vi "PCC_2act_acq.vi"() -> ()   [LabVIEW 2020]
uses:
  C:/Users/quic2/Desktop/DirectUQDLabviewCode/Kinesis/Thorlabs.MotionControl.Controls.dll
  Kinesis/Thorlabs.MotionControl.Controls.dll
  C:/Program Files/Dotfast Consulting/Timetag Explorer 2.26/ttInterface.dll
  Program Files/Dotfast Consulting/Timetag Explorer 2.26/ttInterface.dll
  C:/Users/quic2/Desktop/DirectUQDLabviewCode/Kinesis/ThorLabs.MotionControl.KCube.DCServoCLI.dll
  Kinesis/ThorLabs.MotionControl.KCube.DCServoCLI.dll
  C:/Users/quic2/Desktop/DirectUQDLabviewCode/Kinesis/Thorlabs.MotionControl.KCube.StepperMotorCLI.dll
  Kinesis/Thorlabs.MotionControl.KCube.StepperMotorCLI.dll
  <vilib>/Utility/file.llb/Write Delimited Spreadsheet (string).vi
panel:
  out "x*y":i32=524580565 format="%.3p"
  out "Header":string[](array[string])=["Time Counter (5ns)", "R", "S1", "S2", "RvS1b", "RvS1p", "RvS2b", "RvS2p", "S1pvS2p", "S1bvS2b", "S1bvS2p", "S1pvS2b", "RvS1pvS2p", "RvS1bvS2b"]
  out "R Singles\n Rate (Hz)":u32=294126 format="%.2p"
  out "Horizontal S1\n singles Rate (Hz)":u32=5 format="%.2p"
  out "Vertical S2 \nSingles Rate (Hz)":u32=5 format="%.2p"
  in  "Repetitions":i32=5
  in  "Acquisition \nTime (s)":dbl=0.5
  in  "V  Zero Error":dbl=7.0 format="%#_13g"
  in  "H Zero Error":dbl=7.5 format="%#_13g"
  in  "HWP_ZeroError":dbl=15.0 format="%#_13g"
  out "Current HWP Angle":dbl=15.0
  out "V centroid Singles":dbl=6.986141506451791
  out "H centroid Singles":dbl=7.447438431946241
  out "V Singles":dbl=6.950874322723666 format="%.4e"
  out "H Singles":dbl=7.7419281256167665 format="%.4e"
  in  "Folder":path=path "D:/PCC/2021/3_March/directUQD/6thMarch/RawFileTest/Test5"
  in  "# of Beam Scan":i32=1
  out "V Position":dbl=7.25
  out "H Position":dbl=9.0
  in  "stop":bool
  out "HWP #Iterations":dbl
  out "V # Iterations":dbl=60.0
  out "H #Iterations":dbl=60.0
  in  "HWP_ Stop":dbl=20.0 min=0.0 max=359.0
  in  "HWP_Step":dbl=10.0 min=1e-05 max=359.0
  in  "V Final Position":dbl=7.25 min=0.0 max=25.0
  in  "V Step":dbl=0.05 min=1e-10 max=15.0
  in  "H Final Position":dbl=9.0 min=0.0 max=25.0
  in  "H Step":dbl=0.05 min=1e-10 max=15.0
  in  "V Initial Position":dbl=4.0 min=0.0 max=25.0
  in  "HWP_Start":dbl=15.0 min=0.0 max=359.0
  in  "HWP_post":refnum<k24>(container)
  in  "H Initial Position":dbl=5.75 min=0.0 max=25.0
  in  "Actuator Vertical":refnum<k24>(container)
  in  "Actuator Horizontal":refnum<k24>(container)
  out "Waveform Chart":T1(graph)
  out "Time per Pos":dbl=2.5
  out "Array":i32[](array[numeric])=[844176, 4, 12, 0, 0, 0, 0, 0, 0, 0, 0, 0, 0]
  in  "Ctw(ns)":dbl=2.0
  in  "S2b":u8=10
  in  "S2p":u8=9
  in  "S1b":u8=8
  in  "S1p":u8=7
  in  "R":u8=5
  in  "Ch Array":u8[](array[numeric])=[5, 7, 8, 9, 10] caption="Ch"
  in  "Ch Delay (ns)":dbl[](array[numeric])=[120.0, 11.0, 86.0, 7.5, 82.5]
  # "FOLDER PATH"
  # "HORIZONTAL ACTUATOR"
  # "VERTICAL ACTUATOR"
  # "POST-SELECTION HWP"
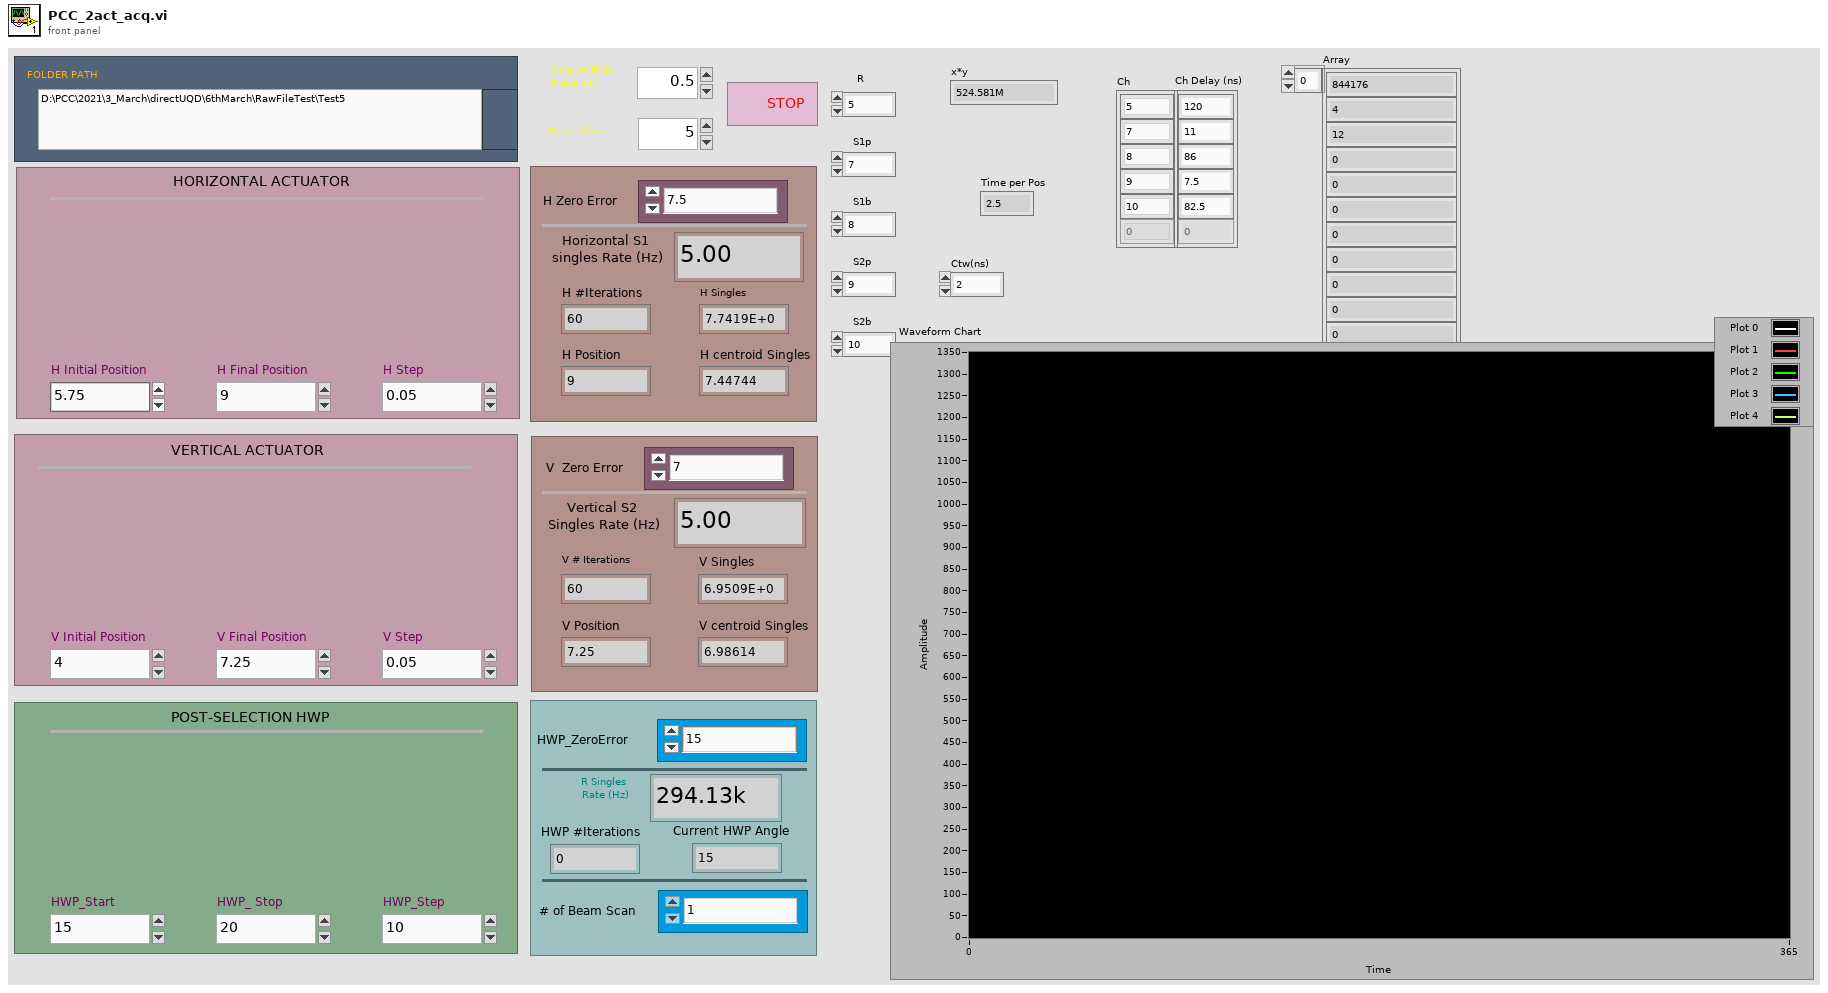
[diagram p1: front panel]
types:
  T1 = cluster{"[0]":dbl, "[1]":dbl, "[2]":dbl, "[3]":dbl, "[4]":dbl, "[5]":dbl, "[6]":dbl, "[7]":dbl, "[8]":dbl}
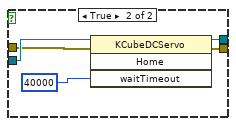
[diagram p3: hidden frame]
diagram:
  # "We want 3 singles\n4 coincidences(peak)\n4 coincidences(BG)\n\nLogic 16 channels\nWe neeed 4+4+3 =11\n\n\nLogic has no per ch delay\nThey must be added in physical channel\n\nSo we need at least 5 physical Chanel\n1 for ref (100)\n1 for H S (delay for peak, 5 )\n1 for HS (delay BG, 75)\n(split the sma into 2 anc connect\nSame signal in both channels)"
  n1 = flat-sequence {
    tunnel: [w110] -> w30
    tunnel: [w109] -> w29
    tunnel: w30 -> [w125]
    tunnel: w29 -> [w124]
    tunnel: [w132] -> w86
    tunnel: [w131] -> w85
    tunnel: [w130] -> w78
    tunnel: [w129] -> w77
    tunnel: w86 -> [w154]
    tunnel: w85 -> [w153]
    tunnel: [w154] -> w83
    tunnel: [w153] -> w81
    tunnel: [w152] -> w79
    tunnel: w78 -> [w151]
    tunnel: w77 -> [w150]
    tunnel: [w151] -> w70
    tunnel: [w150] -> w63
    tunnel: [w149] -> w60
    tunnel: [w148] -> w59
    tunnel: [w147] -> w19
    tunnel: [w181] -> w84
    tunnel: w83 -> [w181]
    tunnel: [w180] -> w82
    tunnel: w81 -> [w180]
    tunnel: [w179] -> w80
    tunnel: w79 -> [w179]
    tunnel: [w178] -> w71
    tunnel: w70 -> [w178]
    tunnel: [w177] -> w64
    tunnel: w63 -> [w177]
    tunnel: w60 -> [w176]
    tunnel: w59 -> [w175]
    tunnel: [w176] -> w53
    tunnel: [w175] -> w45
    tunnel: [w174] -> w38
    tunnel: [w173] -> w31
    tunnel: [w172] -> w20
    tunnel: w19 -> [w172]
    tunnel: [w171] -> w18
    tunnel: [w170] -> w17
    tunnel: [w209] -> w108
    tunnel: [w211] -> w107
    tunnel: [w210] -> w106
    tunnel: [w209] -> w92
    tunnel: w84 -> [w202]
    tunnel: w82 -> [w201]
    tunnel: w80 -> [w200]
    tunnel: [w208] -> w72
    tunnel: w71 -> [w208]
    tunnel: [w207] -> w65
    tunnel: w64 -> [w207]
    tunnel: [w206] -> w54
    tunnel: w53 -> [w206]
    tunnel: [w205] -> w46
    tunnel: w45 -> [w205]
    tunnel: [w204] -> w39
    tunnel: w38 -> [w204]
    tunnel: [w203] -> w32
    tunnel: w31 -> [w203]
    tunnel: [w202] -> w27
    tunnel: [w201] -> w25
    tunnel: w20 -> [w199]
    tunnel: w18 -> [w198]
    tunnel: w17 -> [w197]
    tunnel: [w200] -> w15
    tunnel: [w199] -> w13
    tunnel: [w198] -> w11
    tunnel: [w197] -> w9
    tunnel: w108 -> [w247]
    tunnel: w107 -> [w246]
    tunnel: w106 -> [w231]
    tunnel: [w236] -> w105
    tunnel: [w235] -> w104
    tunnel: [w230] -> w99
    tunnel: w92 -> [w229]
    tunnel: [w229] -> w91
    tunnel: [w228] -> w73
    tunnel: w72 -> [w228]
    tunnel: [w227] -> w66
    tunnel: w65 -> [w227]
    tunnel: [w226] -> w55
    tunnel: w54 -> [w226]
    tunnel: [w225] -> w47
    tunnel: w46 -> [w225]
    tunnel: [w224] -> w40
    tunnel: w39 -> [w224]
    tunnel: [w223] -> w33
    tunnel: w32 -> [w223]
    tunnel: [w222] -> w28
    tunnel: w27 -> [w222]
    tunnel: [w221] -> w26
    tunnel: w25 -> [w221]
    tunnel: [w220] -> w16
    tunnel: w15 -> [w220]
    tunnel: [w219] -> w14
    tunnel: w13 -> [w219]
    tunnel: [w218] -> w12
    tunnel: w11 -> [w218]
    tunnel: [w217] -> w10
    tunnel: w9 -> [w217]
    tunnel: w105 -> [w272]
    tunnel: w104 -> [w271]
    tunnel: [w272] -> w103
    tunnel: [w271] -> w102
    tunnel: [w270] -> w101
    tunnel: [w269] -> w100
    tunnel: w99 -> [w269]
    tunnel: w91 -> [w268]
    tunnel: [w268] -> w90
    tunnel: [w267] -> w74
    tunnel: w73 -> [w267]
    tunnel: [w266] -> w67
    tunnel: w66 -> [w266]
    tunnel: [w265] -> w56
    tunnel: w55 -> [w265]
    tunnel: [w264] -> w48
    tunnel: w47 -> [w264]
    tunnel: [w263] -> w41
    tunnel: w40 -> [w263]
    tunnel: [w262] -> w34
    tunnel: w33 -> [w262]
    tunnel: w28 -> [w261]
    tunnel: w26 -> [w260]
    tunnel: [w261] -> w23
    tunnel: [w260] -> w21
    tunnel: w16 -> [w257]
    tunnel: w14 -> [w256]
    tunnel: w12 -> [w259]
    tunnel: w10 -> [w258]
    tunnel: [w259] -> w7
    tunnel: [w258] -> w5
    tunnel: [w257] -> w3
    tunnel: [w256] -> w1
    tunnel: w103 -> [w328]
    tunnel: w102 -> [w327]
    tunnel: w101 -> [w329]
    tunnel: w100 -> [w326]
    tunnel: [w329] -> w98
    tunnel: [w321] -> w97
    tunnel: [w320] -> w96
    tunnel: [w305] -> w95
    tunnel: w90 -> [w319]
    tunnel: [w319] -> w89
    tunnel: [w304] -> w87
    tunnel: [w317] -> w75
    tunnel: w74 -> [w317]
    tunnel: [w316] -> w68
    tunnel: w67 -> [w316]
    tunnel: [w315] -> w57
    tunnel: w56 -> [w315]
    tunnel: [w314] -> w49
    tunnel: w48 -> [w314]
    tunnel: [w313] -> w42
    tunnel: w41 -> [w313]
    tunnel: [w312] -> w35
    tunnel: w34 -> [w312]
    tunnel: [w311] -> w24
    tunnel: w23 -> [w311]
    tunnel: [w310] -> w22
    tunnel: w21 -> [w310]
    tunnel: [w309] -> w8
    tunnel: w7 -> [w309]
    tunnel: [w308] -> w6
    tunnel: w5 -> [w308]
    tunnel: [w307] -> w4
    tunnel: w3 -> [w307]
    tunnel: [w306] -> w2
    tunnel: w1 -> [w306]
    tunnel: w98 -> [w347]
    tunnel: w97 -> [w349]
    tunnel: w96 -> [w348]
    tunnel: w95 -> [w346]
    tunnel: [w345] -> w94
    tunnel: [w344] -> w93
    tunnel: w89 -> [w343]
    tunnel: [w343] -> w88
    tunnel: w87 -> [w342]
    tunnel: [w341] -> w76
    tunnel: w75 -> [w341]
    tunnel: [w340] -> w69
    tunnel: w68 -> [w340]
    tunnel: [w339] -> w58
    tunnel: w57 -> [w339]
    tunnel: [w338] -> w50
    tunnel: w49 -> [w338]
    tunnel: [w337] -> w43
    tunnel: w42 -> [w337]
    tunnel: [w336] -> w36
    tunnel: w35 -> [w336]
    tunnel: w24 -> [w335]
    tunnel: w22 -> [w334]
    tunnel: w8 -> [w333]
    tunnel: w6 -> [w332]
    tunnel: w4 -> [w331]
    tunnel: w2 -> [w330]
    tunnel: w94 -> [w608]
    tunnel: w93 -> [w607]
    tunnel: w88 -> [w606]
    tunnel: w76 -> [w604]
    tunnel: w69 -> [w603]
    tunnel: [w604] -> w62
    tunnel: [w603] -> w61
    tunnel: w58 -> [w602]
    tunnel: [w602] -> w52
    tunnel: [w601] -> w51
    tunnel: w50 -> [w601]
    tunnel: [w600] -> w44
    tunnel: w43 -> [w600]
    tunnel: [w599] -> w37
    tunnel: w36 -> [w599]
    tunnel: w62 -> [w612]
    tunnel: w61 -> [w609]
    tunnel: w52 -> [w616]
    tunnel: w51 -> [w613]
    tunnel: w44 -> [w618]
    tunnel: w37 -> [w617]
    frame #0 {
    }
    frame #1 {
      # "Calculate Iterations"
      n2 = local read "V Initial Position"() -> (w113:dbl)
      n3 = local read "V Final Position"() -> (w114:dbl)
      n4 = local read "H Initial Position"() -> (w117:dbl)
      n5 = local read "H Final Position"() -> (w118:dbl)
      n6 = local read "V Step"() -> (w111:dbl)
      n7 = local read "HWP_ Stop"() -> (w123:dbl)
      n8 = local read "HWP_Step"() -> (w120:dbl)
      n9 = local read "H Step"() -> (w116:dbl)
      n10 = local read "HWP_Start"() -> (w122:dbl)
      n11 = Subtract(x=w123, y=w122) -> (x-y=w121:dbl)
      n12 = Subtract(x=w114, y=w113) -> (x-y=w112:dbl)
      n13 = Subtract(x=w118, y=w117) -> (x-y=w115:dbl)
      n14 = Quotient & Remainder(x=w121, y=w120) -> (floor(x/y)=w119:dbl)  [unwired: 1 out]
      n15 = Quotient & Remainder(x=w112, y=w111) -> (floor(x/y)=w109:dbl)  [unwired: 1 out]
      n16 = Quotient & Remainder(x=w115, y=w116) -> (floor(x/y)=w110:dbl)  [unwired: 1 out]
      n17 = local write "HWP #Iterations"(w119) -> ()
      n18 = local write "V # Iterations"(w109) -> ()
      n19 = local write "H #Iterations"(w110) -> ()
    }
    frame #2 {
      # "Check if # iterations are same for H and V actuators"
      n20 = Not Equal?(x=w125, y=w124) -> (x != y?=w126:bool)
      n21 = case shown="True" w126 {
        frame False {
        }
        frame True {
          n22 = call "Display Message to User"() -> ("OK"=w127:bool)  [unwired: 10 in, 1 out]
          n23 = Stop(stop? (T)=w127) -> ()
        }
      }
    }
    frame #3 {
      # "Create HWP_post"
      n24 = property class="KCubeDCServoControl"(reference="HWP_post", "SerialNumber"="27503775") -> (reference out=w138:refnum<k24>, error out=w137:errorcluster)  [unwired: 1 in]
      n25 = invoke class="KCubeDCServoControl" method="CreateDevice"(reference=w138, error in=w137) -> (reference out=w135:refnum<k24>, error out=w136:errorcluster)  [unwired: 1 in, 1 out]
      n26 = property class="KCubeDCServoControl"(reference=w135, error in=w136) -> (reference out=w130:refnum<k24>, error out=w129:errorcluster, "Device"=w134:refnum<k24>)
      n27 = case shown="False" FALSE {
        tunnel: w134 -> [w141 w146]
        tunnel: [w141 w144] -> w132
        tunnel: [w140 w143] -> w131
        tunnel: w129 -> [w140 w142]
        frame False {
        }
        frame True {
          n28 = invoke class="KCubeDCServo" method="Home"(reference=w146, error in=w142, "waitTimeout"=40000) -> (reference out=w144:refnum<k24>, error out=w143:errorcluster)  [unwired: 1 in, 2 out]
        }
      }
    }
    frame #4 {
      # "Create H-Actuator"
      n29 = property class="KCubeStepperControl"(reference="Actuator Horizontal", "SerialNumber"="26002814") -> (reference out=w158:refnum<k24>, error out=w159:errorcluster)  [unwired: 1 in]
      n30 = invoke class="KCubeStepperControl" method="CreateDevice"(reference=w158, error in=w159) -> (reference out=w161:refnum<k24>, error out=w160:errorcluster)  [unwired: 1 in, 1 out]
      n31 = property class="KCubeStepperControl"(reference=w161, error in=w160) -> (reference out=w149:refnum<k24>, error out=w148:errorcluster, "Device"=w162:refnum<k24>)
      n32 = case shown="True" FALSE {
        tunnel: w162 -> [w164 w169]
        tunnel: w148 -> [w163 w167]
        tunnel: [w163 w166] -> w147
        tunnel: [w164 w165] -> w152
        frame False {
        }
        frame True {
          n33 = invoke class="KCubeStepper" method="Home"(reference=w169, error in=w167, "waitTimeout"=36000) -> (reference out=w165:refnum<k24>, error out=w166:errorcluster)  [unwired: 1 in, 2 out]
        }
      }
    }
    frame #5 {
      # "Create V-Actuator"
      n34 = property class="KCubeStepperControl"(reference="Actuator Vertical", "SerialNumber"="26001200") -> (reference out=w189:refnum<k24>, error out=w188:errorcluster)  [unwired: 1 in]
      n35 = invoke class="KCubeStepperControl" method="CreateDevice"(reference=w189, error in=w188) -> (reference out=w186:refnum<k24>, error out=w187:errorcluster)  [unwired: 1 in, 1 out]
      n36 = property class="KCubeStepperControl"(reference=w186, error in=w187) -> (reference out=w174:refnum<k24>, error out=w173:errorcluster, "Device"=w185:refnum<k24>)
      n37 = case shown="True" FALSE {
        tunnel: w185 -> [w191 w196]
        tunnel: w173 -> [w190 w194]
        tunnel: [w190 w193] -> w170
        tunnel: [w191 w192] -> w171
        frame False {
        }
        frame True {
          n38 = invoke class="KCubeStepper" method="Home"(reference=w196, error in=w194, "waitTimeout"=36000) -> (reference out=w192:refnum<k24>, error out=w193:errorcluster)  [unwired: 1 in, 2 out]
        }
      }
    }
    frame #6 {
      # "Create UQD TimeTag Interface"
      n39 = constructor class="TTInterface"() -> (reference out=w216:refnum<k24>, error out=w215:errorcluster)  [unwired: 3 in, 1 out]
      n40 = invoke class="TTInterface" method="Open"(reference=w216, error in=w215, "nr"=1) -> (reference out=w212:refnum<k24>, error out=w213:errorcluster)  [unwired: 1 in, 2 out]
      n41 = invoke class="TTInterface" method="GetResolution"(reference=w212, error in=w213) -> (reference out=w209:refnum<k24>, error out=w211:errorcluster, "GetResolution"=w210:dbl)  [unwired: 1 in]
    }
    frame #7 {
      # "Set Channel delays"
      # "Create UQD Logic"
      n42 = constructor class="Logic"(error in=w246, "tti"=w247) -> (reference out=w245:refnum<k24>, error out=w244:errorcluster)  [unwired: 2 in, 2 out]
      n43 = invoke class="Logic" method="SwitchLogicMode"(reference=w245, error in=w244) -> (reference out=w243:refnum<k24>, error out=w242:errorcluster)  [unwired: 1 in, 1 out]
      n44 = Multiply(x="Ctw(ns)", y=1e-09) -> (x*y=w232:dbl)
      n45 = Multiply(x="Ch Delay (ns)", y=1e-09) -> (x*y=w239:dbl[])
      n46 = Divide(x=w239, y=w231) -> (x/y=w238:dbl[])
      n47 = Divide(x=w232, y=w231) -> (x/y=w230:dbl)
      n48 = for {
        tunnel: w243 -> [w253]
        tunnel: w242 -> [w252]
        tunnel: w238 -> [w251] mode=indexing
        tunnel: "Ch Array" -> [w250] mode=indexing
        tunnel: [w249] -> w236
        tunnel: [w248] -> w235
        n49 = invoke class="Logic" method="SetDelay"(reference=w253, error in=w252, "input"=w250, "delay"=w251) -> (reference out=w249:refnum<k24>, error out=w248:errorcluster)  [unwired: 1 in, 3 out]
      }
    }
    frame #8 {
      # "Createing Array for different coincidence patterns"
      n50 = Build Array("Time Counter (5ns)" ("string"), "R" ("string"), "S1" ("string"), "S2" ("string"), "RvS1b" ("string"), "RvS1p" ("string"), "RvS2b" ("string"), "RvS2p" ("string"), "S1pvS2p" ("string"), "S1bvS2b" ("string"), "S1bvS2p" ("string"), "S1pvS2b" ("string"), "RvS1pvS2p" ("string"), "RvS1bvS2b" ("string")) -> (→"Header":string[])
      n51 = Build Array("R") -> (w277:u8[])
      n52 = Build Array("S1p") -> (w275:u8[])
      n53 = Build Array("S2p") -> (w273:u8[])
      n54 = Build Array("R", "S1b") -> (w291:u8[])
      n55 = Build Array("R", "S1p") -> (w290:u8[])
      n56 = Build Array("R", "S2b") -> (w289:u8[])
      n57 = Build Array("R", "S2p") -> (w288:u8[])
      n58 = Build Array("S1p", "S2p") -> (w287:u8[])
      n59 = Build Array("S1b", "S2b") -> (w286:u8[])
      n60 = Build Array("S1b", "S2p") -> (w285:u8[])
      n61 = Build Array("S1p", "S2b") -> (w284:u8[])
      n62 = Build Array("R", "S1p", "S2p") -> (w283:u8[])
      n63 = Build Array("R", "S1b", "S2b") -> (w282:u8[])
      n64 = Build Array(w277, w275, w273, w291, w290, w289, w288, w287, w286, w285, w284, w283, w282) -> (w270:u8[][])
    }
    frame #9 {
      # "Set CTW and ACQ time"
      n65 = local read "Acquisition \nTime (s)"() -> (w305:dbl)
      n66 = invoke class="Logic" method="SetWindowWidth"(reference=w328, error in=w327, "window"=w326) -> (reference out=w323:refnum<k24>, error out=w324:errorcluster)  [unwired: 1 in, 2 out]
      n67 = local read "Repetitions"() -> (w304:i32)
      n68 = call "Time Delay"("error in (no error)"=w324, "Delay Time (s)"=0.1) -> ("error out"=w322:errorcluster)  [unwired: 9 in]
      n69 = Multiply(x=w305, y=w304) -> (x*y=→"Time per Pos":dbl)
      n70 = invoke class="Logic" method="ReadLogic"(reference=w323, error in=w322) -> (reference out=w321:refnum<k24>, error out=w320:errorcluster)  [unwired: 1 in, 1 out]
    }
    frame #10 {
      n71 = while {
        tunnel: w347 -> [w369]
        tunnel: w346 -> [w368]
        tunnel: w342 -> [w365]
        shift-right: [w367] -> w345
        shift-left: w349 -> [w371]
        shift-right: [w366] -> w344
        shift-left: w348 -> [w370]
        tunnel: w335 -> [w364]
        tunnel: w334 -> [w363]
        tunnel: w333 -> [w357]
        tunnel: w332 -> [w355]
        tunnel: w331 -> [w353]
        tunnel: w330 -> [w351]
        i -> [w350]
        stop <- w359 stop-if-true
        # "Loop Over HWP angle"
        n72 = flat-sequence {
          tunnel: w365 -> [w396]
          tunnel: w368 -> [w397]
          tunnel: w369 -> [w398]
          tunnel: w370 -> [w399]
          tunnel: w371 -> [w400]
          tunnel: [w400] -> w380
          tunnel: [w399] -> w379
          tunnel: [w398] -> w378
          tunnel: [w397] -> w377
          tunnel: [w396] -> w376
          tunnel: w364 -> [w394]
          tunnel: w363 -> [w393]
          tunnel: w350 -> [w390]
          tunnel: [w387] -> w358
          tunnel: w357 -> [w387]
          tunnel: [w386] -> w356
          tunnel: w355 -> [w386]
          tunnel: [w385] -> w354
          tunnel: w353 -> [w385]
          tunnel: [w384] -> w352
          tunnel: w351 -> [w384]
          tunnel: [w408] -> w375
          tunnel: [w407] -> w374
          tunnel: w380 -> [w412]
          tunnel: w379 -> [w411]
          tunnel: w378 -> [w410]
          tunnel: w377 -> [w409]
          tunnel: w376 -> [w406]
          tunnel: w358 -> [w405]
          tunnel: w356 -> [w404]
          tunnel: w354 -> [w403]
          tunnel: w352 -> [w402]
          tunnel: w350 -> [w401]
          tunnel: w375 -> [w596]
          tunnel: [w596] -> w373
          tunnel: w374 -> [w595]
          tunnel: [w595] -> w372
          tunnel: [w597] -> w366
          tunnel: [w598] -> w367
          tunnel: w373 -> [w598]
          tunnel: w372 -> [w597]
          frame #0 {
            # "Rotate HWP"
            n73 = local read "HWP_Step"() -> (w391:dbl)
            n74 = local read "HWP_Start"() -> (w392:dbl)
            n75 = Multiply(x=w391, y=w390) -> (x*y=w389:dbl)
            n76 = Add(x=w392, y=w389) -> (x+y=w388:dbl)
            n77 = invoke class="KCubeDCServo" method="MoveTo"(reference=w394, error in=w393, "position"=w388, "waitTimeout"=40000) -> (reference out=w383:refnum<k24>, error out=w382:errorcluster)  [unwired: 1 in, 3 out]
            n78 = property class="KCubeDCServo"(reference=w383, error in=w382) -> ("Position"=w381:dbl)  [unwired: 2 out]
            n79 = local write "Current HWP Angle"(w381) -> ()
          }
          frame #1 {
            n80 = while {
              tunnel: w410 -> [w426]
              tunnel: w409 -> [w425]
              tunnel: w406 -> [w422]
              tunnel: w405 -> [w421]
              tunnel: w404 -> [w420]
              tunnel: w403 -> [w419]
              tunnel: w402 -> [w418]
              shift-right: [w424] -> w408
              shift-left: w412 -> [w428]
              shift-right: [w423] -> w407
              shift-left: w411 -> [w427]
              tunnel: w401 -> [w414]
              i -> [w417]
              stop <- w415 stop-if-true
              n81 = flat-sequence {
                tunnel: w428 -> [w441]
                tunnel: w427 -> [w440]
                tunnel: w426 -> [w439]
                tunnel: w425 -> [w438]
                tunnel: [w437] -> w424
                tunnel: [w436] -> w423
                tunnel: w422 -> [w435]
                tunnel: w421 -> [w434]
                tunnel: w420 -> [w433]
                tunnel: w419 -> [w432]
                tunnel: w418 -> [w431]
                tunnel: w414 -> [w430]
                tunnel: w413 -> [w429]
                frame #0 {
                  n82 = while {
                    tunnel: w439 -> [w461]
                    tunnel: w438 -> [w460]
                    tunnel: w435 -> [w457]
                    shift-right: [w459] -> w437
                    shift-left: w441 -> [w463]
                    shift-right: [w458] -> w436
                    shift-left: w440 -> [w462]
                    tunnel: w434 -> [w456]
                    tunnel: w433 -> [w455]
                    tunnel: w432 -> [w454]
                    tunnel: w431 -> [w453]
                    tunnel: [w442] -> _
                    tunnel: w430 -> [w444]
                    tunnel: w429 -> [w443]
                    i -> [w442]
                    stop <- w446 stop-if-true
                    # "Loop over actuators"
                    n83 = flat-sequence {
                      tunnel: w457 -> [w490]
                      tunnel: w460 -> [w491]
                      tunnel: w461 -> [w492]
                      tunnel: w462 -> [w493]
                      tunnel: w463 -> [w494]
                      tunnel: [w494] -> w470
                      tunnel: [w493] -> w469
                      tunnel: [w492] -> w468
                      tunnel: [w491] -> w467
                      tunnel: [w490] -> w466
                      tunnel: w456 -> [w489]
                      tunnel: w455 -> [w488]
                      tunnel: w454 -> [w474]
                      tunnel: w453 -> [w473]
                      tunnel: [w482] -> _
                      tunnel: w442 -> [w482]
                      tunnel: [w477] -> w452
                      tunnel: [w476] -> w451
                      tunnel: [w475] -> w450
                      tunnel: w470 -> [w498]
                      tunnel: w469 -> [w496]
                      tunnel: w468 -> [w510]
                      tunnel: w467 -> [w509]
                      tunnel: w466 -> [w506]
                      tunnel: [w508] -> w465
                      tunnel: [w507] -> w464
                      tunnel: w452 -> [w505]
                      tunnel: w451 -> [w504]
                      tunnel: w450 -> [w502]
                      tunnel: [w499] -> w445
                      tunnel: [w593] -> w458
                      tunnel: [w594] -> w459
                      tunnel: w465 -> [w594]
                      tunnel: w464 -> [w593]
                      tunnel: w445 -> [w591]
                      tunnel: w444 -> [w586]
                      tunnel: w443 -> [w583]
                      tunnel: w442 -> [w585]
                      frame #0 {
                        w483 = 40000 ("waitTimeout")
                        # "Move Actuators"
                        n84 = local read "V Initial Position"() -> (w487:dbl)
                        n85 = local read "V Step"() -> (w486:dbl)
                        n86 = local read "H Initial Position"() -> (w480:dbl)
                        n87 = Multiply(x=w486, y=w482) -> (x*y=w485:dbl)
                        n88 = local read "H Step"() -> (w481:dbl)
                        n89 = Add(x=w487, y=w485) -> (x+y=w484:dbl)
                        n90 = invoke class="KCubeStepper" method="MoveTo"(reference=w489, error in=w488, "position"=w484, "waitTimeout"=w483) -> (reference out=w477:refnum<k24>, error out=w472:errorcluster)  [unwired: 1 in, 3 out]
                        n91 = Multiply(x=w481, y=w482) -> (x*y=w479:dbl)
                        n92 = Add(x=w480, y=w479) -> (x+y=w478:dbl)
                        n93 = Merge Errors(w473, w472) -> (w471:errorcluster)
                        n94 = invoke class="KCubeStepper" method="MoveTo"(reference=w474, error in=w471, "position"=w478, "waitTimeout"=w483) -> (reference out=w475:refnum<k24>, error out=w476:errorcluster)  [unwired: 1 in, 3 out]
                      }
                      frame #1 {
                        n95 = invoke class="Logic" method="ReadLogic"(reference=w498, error in=w496) -> (reference out=w497:refnum<k24>, error out=w495:errorcluster)  [unwired: 1 in, 1 out]
                        n96 = property class="KCubeStepper"(reference=w505, error in=w504) -> (error out=w503:errorcluster, "Position"=w500:dbl)  [unwired: 1 out]
                        n97 = while {
                          tunnel: w510 -> [w525]
                          tunnel: w509 -> [w524]
                          shift-right: [w523] -> w508
                          shift-left: w497 -> [w527]
                          shift-right: [w522] -> w507
                          shift-left: w495 -> [w526]
                          tunnel: w506 -> [w519]
                          tunnel: [w514] -> w499 mode=indexing
                          i -> [w521]
                          stop <- w518 stop-if-true
                          n98 = flat-sequence {
                            tunnel: w527 -> [w541]
                            tunnel: w526 -> [w542]
                            tunnel: w525 -> [w537]
                            tunnel: w524 -> [w543]
                            tunnel: [w534] -> w530
                            tunnel: [w533] -> w529
                            tunnel: [w532] -> w528
                            tunnel: [w531] -> w515
                            tunnel: w530 -> [w567]
                            tunnel: w529 -> [w566]
                            tunnel: w528 -> [w560]
                            tunnel: w515 -> [w563]
                            tunnel: [w567] -> w513
                            tunnel: [w566] -> w512
                            tunnel: [w564] -> w511
                            tunnel: [w572] -> w514
                            tunnel: [w568] -> w522
                            tunnel: [w569] -> w523
                            tunnel: w513 -> [w570]
                            tunnel: w512 -> [w571]
                            tunnel: w511 -> [w572]
                            frame #0 {
                              n99 = call "Delay"("error in (no error)"=w542, "Delay Time (s)"=w543) -> ("error out"=w540:errorcluster)  [unwired: 9 in]
                              n100 = invoke class="Logic" method="ReadLogic"(reference=w541, error in=w540) -> (reference out=w539:refnum<k24>, error out=w538:errorcluster)  [unwired: 1 in, 1 out]
                              n101 = invoke class="Logic" method="GetTimeCounter"(reference=w539, error in=w538) -> (reference out=w536:refnum<k24>, error out=w535:errorcluster, "GetTimeCounter"=w531:i32)  [unwired: 1 in]
                              n102 = for {
                                tunnel: w537 -> [w553] mode=indexing
                                tunnel: w536 -> [w549]
                                tunnel: w535 -> [w548]
                                tunnel: [w547] -> w534
                                tunnel: [w546] -> w533
                                tunnel: [w545] -> w532 mode=indexing
                                n103 = Decrement(x=w553) -> (x-1=w552:u8[])
                                n104 = for {
                                tunnel: w552 -> [w555] mode=indexing
                                tunnel: [w554] -> w551 mode=indexing
                                n105 = Scale By Power Of 2(n=w555, x=1) -> (x*2^n=w554:i32)
                                }
                                n106 = Add Array Elements(numeric array=w551) -> (sum=w550:i32)
                                n107 = invoke class="Logic" method="CalcCount"(reference=w549, error in=w548, "pos"=w550, "neg"=0) -> (reference out=w547:refnum<k24>, error out=w546:errorcluster, "CalcCount"=w545:i32)  [unwired: 1 in, 2 out]
                              }
                            }
                            frame #1 {
                              # "5 ns"
                              n108 = Build Array (concatenate)(w563, w560) -> (w564:i32[])
                              n109 = Multiply(x=w563, y=5) -> (x*y=w558:i32)
                              "x*y" <- w558
                              n110 = Multiply(x=1e-09, y=w558) -> (x*y=w557:dbl)
                              n111 = Divide(x=w560, y=w557) -> (x/y=w561:dbl[])
                              n112 = Array To Cluster(array=w561) -> (cluster=→"Waveform Chart":T1)
                              "Array" <- w560
                            }
                            frame #2 {
                              n113 = invoke class="Logic" method="ReadLogic"(reference=w570, error in=w571) -> (reference out=w569:refnum<k24>, error out=w568:errorcluster)  [unwired: 1 in, 1 out]
                            }
                          }
                          n114 = Increment(x=w521) -> (x+1=w520:i32)
                          n115 = Greater?(x=w520, y=w519) -> (0:w517:bool)
                          n116 = Or(x="stop", y=w517) -> (x .or. y?=w518:bool)
                        }
                        n117 = local write "V Position"(w500) -> ()
                        n118 = property class="KCubeStepper"(reference=w502, error in=w503) -> ("Position"=w501:dbl)  [unwired: 2 out]
                        n119 = local write "H Position"(w501) -> ()
                      }
                      frame #2 {
                        # "ACTPos"
                        # "HWP"
                        # "SAVE RAW DATA"
                        n120 = local read "Header"() -> (w573:string[])
                        n121 = Increment(x=w586) -> (x+1=w584:i32)
                        n122 = Number To Decimal String(number=w584) -> (decimal integer string=w581:string)  [unwired: 1 in]
                        n123 = Number To Decimal String(number=w591) -> (decimal integer string=w592:string[][])  [unwired: 1 in]
                        n124 = local read "Folder"() -> (w588:path)
                        n125 = Build Array (concatenate)(w573, w592) -> (w590:string[][])
                        n126 = Number To Decimal String(number=w583) -> (decimal integer string=w580:string)  [unwired: 1 in]
                        n127 = Increment(x=w585) -> (x+1=w582:i32)
                        n128 = Number To Decimal String(number=w582) -> (decimal integer string=w579:string)  [unwired: 1 in]
                        n129 = Concatenate Strings("HWP" ("string"), w581, "_scan" ("string"), w580, "_pos" ("string"), w579, ".csv" ("string")) -> (w574:string)
                        n130 = Build Path(base path=w588, name or relative path=w574) -> (appended path=w587:path)
                        n131 = call-poly <vilib>:"Write Delimited Spreadsheet.vi"("file path (dialog if empty)"=w587, "2D data"=w590, "delimiter (\\t)"="," ("delimiter (\\t)")) -> ()  [unwired: 11 in, 2 out]
                      }
                    }
                    n132 = local read "H #Iterations"() -> (w449:dbl)
                    n133 = Greater Or Equal?(x=w442, y=w449) -> (x >= y?=w448:bool)
                    n134 = local read "stop"() -> (w447:bool)
                    n135 = Or(x=w448, y=w447) -> (x .or. y?=w446:bool)
                  }
                }
              }
              n136 = local read "# of Beam Scan"() -> (w416:i32)
              n137 = Increment(x=w417) -> (x+1=w413:i32)
              n138 = Greater Or Equal?(x=w413, y=w416) -> (x >= y?=w415:bool)
            }
          }
          frame #2 {
          }
          frame #3 {
          }
        }
        n139 = local read "stop"() -> (w360:bool)
        n140 = local read "HWP #Iterations"() -> (w362:dbl)
        n141 = Greater Or Equal?(x=w350, y=w362) -> (x >= y?=w361:bool)
        n142 = Or(x=w361, y=w360) -> (x .or. y?=w359:bool)
      }
    }
    frame #11 {
      n143 = Close Reference(reference=w608, error in (no error)=w607) -> (error out=w605:errorcluster)
      n144 = invoke class="TTInterface" method="Close"(reference=w606, error in=w605) -> ()  [unwired: 1 in, 3 out]
    }
    frame #12 {
      n145 = invoke class="KCubeStepperControl" method="CloseDevice"(reference=w618, error in=w617) -> (error out=w614:errorcluster)  [unwired: 1 in, 2 out]
      n146 = Merge Errors(w614, w613) -> (w615:errorcluster)
      n147 = invoke class="KCubeStepperControl" method="CloseDevice"(reference=w616, error in=w615) -> (error out=w610:errorcluster)  [unwired: 1 in, 2 out]
      n148 = Merge Errors(w610, w609) -> (w611:errorcluster)
      n149 = invoke class="KCubeDCServoControl" method="CloseDevice"(reference=w612, error in=w611) -> ()  [unwired: 1 in, 3 out]
    }
  }
